vi "runs.list.vi"(8 "error in":errorcluster, 11 "asset in":refnum<class "asset.lvclass">) -> (0 "error out":errorcluster, 2 "Runs":refnum<class "Run.lvclass">[](array[class]), 3 "asset out":refnum<class "asset.lvclass">)   [LabVIEW 2020, in "asset.lvclass"]
uses:
  asset.lvclass
  asset.lvclass/asset.ctl
  Nominal Client/Nominal Client.lvclass
  Run/Run.lvclass
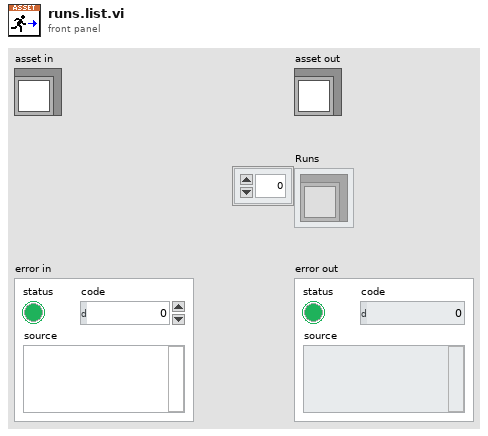
[diagram p1: front panel]
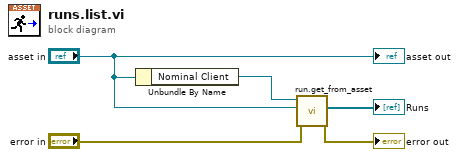
[diagram p0: block diagram]
diagram:
  n1 = Unbundle By Name("asset in") -> ("Nominal Client"=w4:refnum<class "Nominal Client.lvclass">)
  n2 = call "run.get_from_asset.vi"("error in"="error in", "asset"="asset in", "Nominal Client in"=w4) -> ("error out"=→"error out":errorcluster, "Run"=→"Runs":refnum<class "Run.lvclass">[])  [unwired: 6 in, 1 out]
  "asset out" <- "asset in"
